vi "ConvertCSVStringToArray.vi"(11 "CSV String":string="-6.31809e-09, -6.12736e-09, -6.11544e-09, -6.15120e-09, -6.04391e-09, -5.82933e-09, -5.91278e-09, -5.69820e-09, -5.74589e-09, -5.81741e-09\n") -> (3 "Array":dbl[](array[numeric]))   [LabVIEW 2012, in "LV-Utilities.lvlib"]
uses:
  LV-Utilities.lvlib
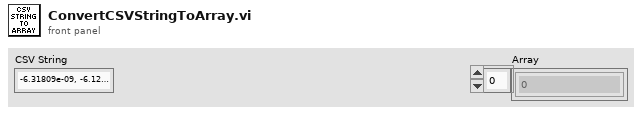
[diagram p1: front panel]
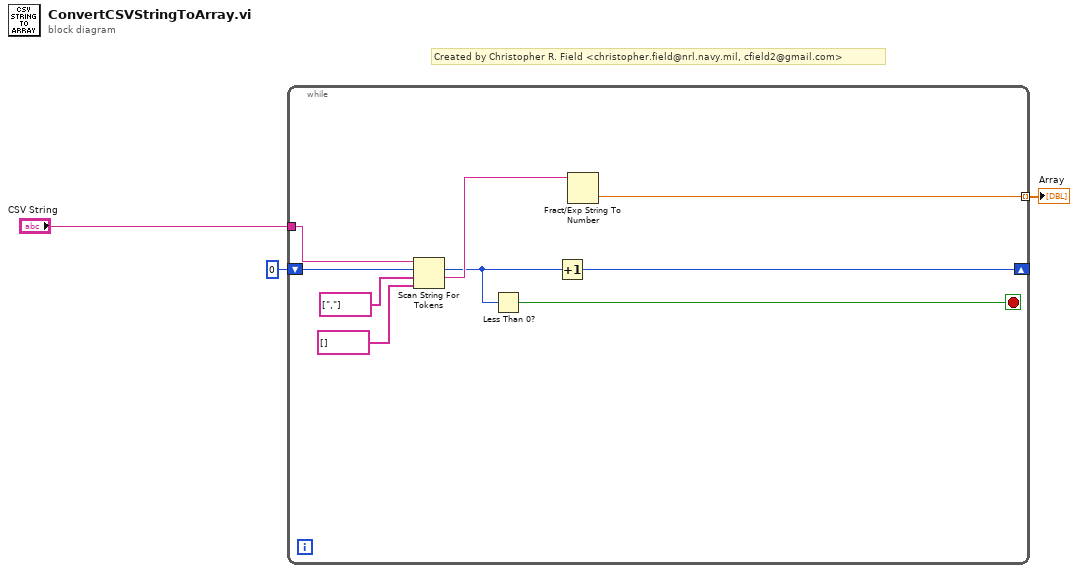
[diagram p0: block diagram]
diagram:
  # "Created by Christopher R. Field <christopher.field@nrl.navy.mil, cfield2@gmail.com>"
  n1 = while {
    tunnel: "CSV String" -> [w12]
    tunnel: [w8] -> w2 mode=indexing
    shift-right: [w4] -> _
    shift-left: 0 ("offset past token") -> [w6]
    stop <- w7 stop-if-true
    n2 = Scan String For Tokens(6:string[] [] ("delimiters (\\s,\\t,\\r,\\n)"), 7:string[] [","] ("operators (none)"), 8:w6, 9:w12) -> (1:w9:string, 2:w5:i32)  [unwired: 2 in, 2 out]
    n3 = Less Than 0?(x=w5) -> (x < 0?=w7:bool)
    n4 = Increment(x=w5) -> (x+1=w4:i32)
    n5 = Fract/Exp String To Number(string=w9) -> (number=w8:dbl)  [unwired: 3 in, 1 out]
  }
  "Array" <- w2
